vi "ConfigureVirtualChannelModule.vi"(8 "error in (no error)":errorcluster) -> (0 "error out":errorcluster, 1 "register data sets":T1[](array[typedef]), 3 "Virtual Channel Config":T4)   [LabVIEW 2017, in "McsaVirtualChannel.lvlib"]
uses:
  <vilib>/addons/InsightCM/Devices/Shared/Mcsa/McsaVirtualChannel/McsaVirtualChannel.lvlib
  <vilib>/addons/InsightCM/Utilities/GlobalConfiguration/GlobalConfiguration.lvlib
  <vilib>/addons/InsightCM/Utilities/DeviceModelHelpers/DeviceModelHelpers.lvlib
  <vilib>/addons/InsightCM/MessageBus/Base/controls/KeyValuePair.ctl
  <vilib>/addons/InsightCM/MessageBus/Base/controls/Tag.ctl
  <vilib>/addons/InsightCM/Devices/Shared/Mcsa/McsaVirtualChannel/controls/VirtualChannel.ctl
  <vilib>/addons/InsightCM/Devices/Shared/Mcsa/McsaVirtualChannel/controls/VirtualChannelGroup.ctl
  <vilib>/addons/InsightCM/Devices/Shared/Mcsa/McsaVirtualChannel/controls/Config.ctl
  <vilib>/addons/InsightCM/MessageBus/Base/controls/DeviceState.ctl
  <vilib>/addons/InsightCM/MessageBus/Base/controls/Condition.ctl
  <vilib>/addons/InsightCM/MessageBus/Base/controls/Trigger.ctl
  <vilib>/addons/InsightCM/MessageBus/Base/controls/OperatingState.ctl
  <vilib>/addons/InsightCM/MessageBus/Base/controls/R2_DataGroup.ctl
  <vilib>/addons/InsightCM/MessageBus/Base/controls/R2_Device.ctl
  <vilib>/addons/InsightCM/MessageBus/Base/controls/R2_Channel.ctl
  <vilib>/addons/InsightCM/MessageBus/Base/controls/R2_DeviceModel.ctl
  <vilib>/addons/InsightCM/MessageBus/Base/controls/Metric.ctl
  <vilib>/addons/InsightCM/MessageBus/Base/controls/BurstModeTrigger.ctl
  <vilib>/addons/InsightCM/Devices/Shared/Mcsa/McsaDataEventCreator/controls/DataSetType.ctl
  <vilib>/addons/InsightCM/Devices/Shared/Mcsa/McsaDataEventCreator/McsaDataEventCreator.lvlib
  <vilib>/addons/InsightCM/Devices/Shared/Mcsa/McsaDataEventCreator/controls/Registry_DataSet.ctl
  <vilib>/addons/InsightCM/Devices/Shared/Mcsa/McsaDataEventCreator/controls/RegisterDataSets.ctl
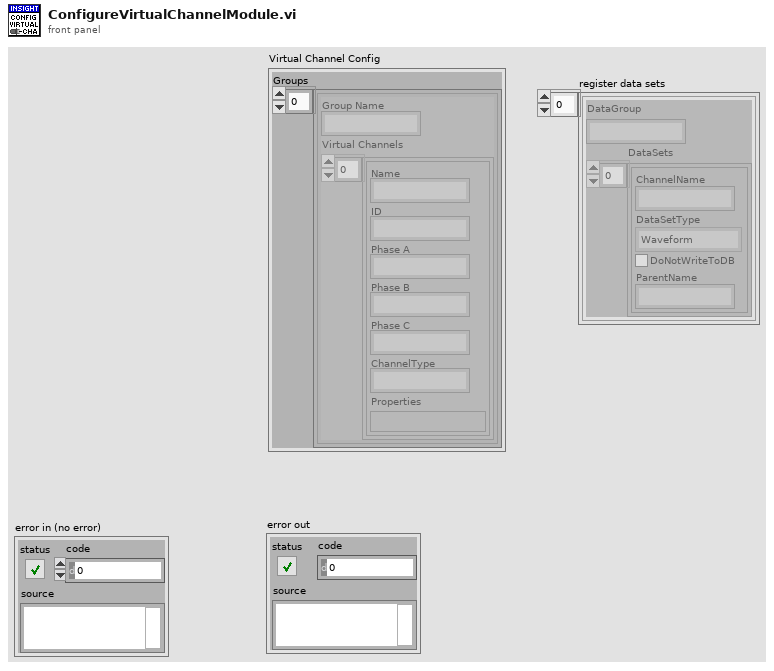
[diagram p1: front panel]
types:
  T1 = typedef "McsaDataEventCreator.lvlib/RegisterDataSets.ctl" = cluster{"DataGroup":string, "DataSets":T2[]}
  T2 = typedef "McsaDataEventCreator.lvlib/Registry_DataSet.ctl" = cluster{"ChannelName":string, "DataSetType":T3, "DoNotWriteToDB":bool, "ParentName":string}
  T3 = typedef "McsaDataEventCreator.lvlib/DataSetType.ctl" = enum16{"Waveform", "MCSAFFT", "TorqueWFM"}
  T4 = typedef "McsaVirtualChannel.lvlib/Config.ctl" = cluster{"Groups":T5[]}
  T5 = typedef "McsaVirtualChannel.lvlib/VirtualChannelGroup.ctl" = cluster{"Group Name":string, "Virtual Channels":T6[]}
  T6 = typedef "McsaVirtualChannel.lvlib/VirtualChannel.ctl" = cluster{"Name":string, "ID":string, "Phase A":string, "Phase B":string, "Phase C":string, "ChannelType":string, "Properties":variant}
  T7 = typedef "R2_DeviceModel.ctl" = cluster{"Device":T8, "Channels":T16[], "Tags":T18[]}
  T8 = typedef "R2_Device.ctl" = cluster{"Id":string, "Name":string, "DeviceType":string, "HardwareName":string, "IpAddress":string, "HardwareInfo":T9[], "ApplicationType":string, "ApplicationVersion":string, "EquipmentIds":string[], "ConfigurationVersion":string, "State":T10, "Properties":T9[], "DataGroups":T11[], "BurstModeTrigger":T15}
  T9 = typedef "KeyValuePair.ctl" = cluster{"Key":string, "Value":string}
  T10 = typedef "DeviceState.ctl" = cluster{"Disabled":bool}
  T11 = typedef "R2_DataGroup.ctl" = cluster{"Name":string, "OperatingStates":T12[], "Properties":T9[], "EquipmentIds":string[], "AssetNodeId":string}
  T12 = typedef "OperatingState.ctl" = cluster{"Name":string, "Properties":T9[], "Triggers":T13[]}
  T13 = typedef "Trigger.ctl" = cluster{"Type":string, "Expression":string, "Conditions":T14[]}
  T14 = typedef "Condition.ctl" = cluster{"Source":string, "Type":string, "Operator":string, "CompareTo":string, "DwellSeconds":dbl}
  T15 = typedef "BurstModeTrigger.ctl" = cluster{"Trigger":T13, "SampleRate":string, "AcquisitionLength":string}
  T16 = typedef "R2_Channel.ctl" = cluster{"Id":string, "DeviceId":string, "Name":string, "ChannelType":string, "HardwareKey":string, "HardwareChannel":string, "DataGroup":string, "Keywords":string[], "EquipmentIds":string[], "Properties":T9[], "Metrics":T17[], "AssetNodeId":string, "MeasType":string, "AssetName":string}
  T17 = typedef "Metric.ctl" = cluster{"Id":string, "Name":string, "Unit":string, "Properties":T9[], "MetricDefinitionInstanceId":string}
  T18 = typedef "Tag.ctl" = cluster{"Id":string, "Path":string, "Name":string, "Datatype":string, "Props":T9[], "Keywords":string[]}
  T19 = typedef "SectionKeyValues.ctl" = cluster{"Section":string, "KeyValues":T9[]}
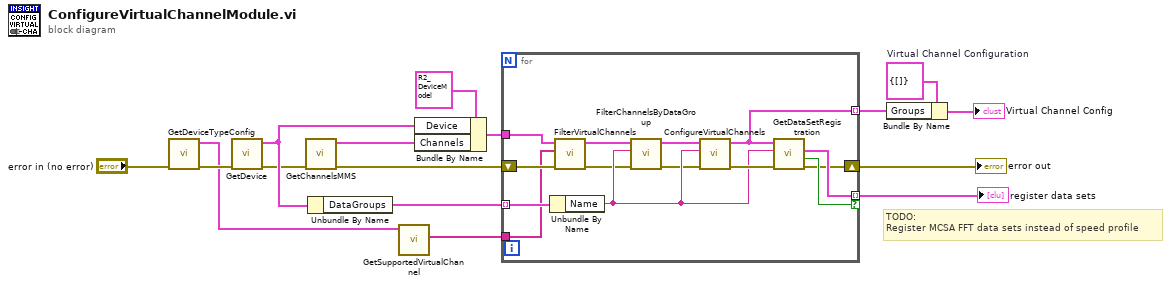
[diagram p0: block diagram]
diagram:
  w8 = T4 {"Groups"=[]}  # Virtual Channel Configuration
  # "TODO:\nRegister MCSA FFT data sets instead of speed profile"
  n1 = call <vilib>:"GetDeviceTypeConfig.vi"("error in (no error)"="error in (no error)") -> ("error out"=w12:errorcluster, "key values"=w7:T19[])  [unwired: 8 in, 1 out]
  n2 = call <vilib>:"GetDevice.vi"("error in (no error)"=w12) -> ("error out"=w1:errorcluster, "device configuration"=w4:T8)  [unwired: 8 in, 1 out]
  n3 = call <vilib>:"GetChannelsMMS.vi"("error in (no error)"=w1) -> ("error out"=w3:errorcluster, "MMS Channels"=w2:T16[])  [unwired: 6 in, 3 out]
  n4 = Unbundle By Name(w4) -> ("DataGroups"=w16:T11[])
  n5 = call <vilib>:"GetSupportedVirtualChannel.vi"("key values"=w7) -> ("not supported virtual channels"=w6:string[])  [unwired: 9 in, 1 out]
  n6 = Bundle By Name(cluster=T7 {"Device"={"Id"="", "Name"="", "DeviceType"="", "HardwareName"="", "IpAddress"="", "HardwareInfo"=[], "ApplicationType"="", "ApplicationVersion"="", "EquipmentIds"=[], "ConfigurationVersion"="", "State"={"Disabled"=FALSE}, "Properties"=[], "DataGroups"=[], "BurstModeTrigger"={"Trigger"={"Type"="", "Expression"="", "Conditions"=[]}, "SampleRate"="", "AcquisitionLength"=""}}, "Channels"=[], "Tags"=[]} ("device model"), "Device"=w4, "Channels"=w2) -> (w9:T7)
  n7 = for {
    shift-right: [w24] -> w15
    shift-left: w3 -> [w21]
    tunnel: w16 -> [w28] mode=indexing
    tunnel: [w29] -> w14 mode=indexing
    tunnel: w6 -> [w19]
    tunnel: w9 -> [w23]
    tunnel: [w26] -> w5 mode=indexing if=w25
    n8 = Unbundle By Name(w28) -> ("Name"=w27:string)
    n9 = call <vilib>:"FilterVirtualChannels.vi"("error in (no error)"=w21, "not supported virtual channels"=w19, "device model"=w23) -> ("error out"=w20:errorcluster, "device model (unsupported virtual channels filtered out)"=w22:T7)  [unwired: 7 in]
    n10 = call <vilib>:"FilterChannelsByDataGroup.vi"("error in (no error)"=w20, "group"=w27, "device model"=w22) -> ("error out"=w17:errorcluster, "channels in data group"=w18:T16[])  [unwired: 7 in]
    n11 = call <vilib>:"ConfigureVirtualChannels.vi"("error in (no error)"=w17, "data group name"=w27, "channels in this group"=w18) -> ("error out"=w30:errorcluster, "virtual channel config"=w29:T5)  [unwired: 6 in, 1 out]
    n12 = call <vilib>:"GetDataSetRegistration.vi"("error in (no error)"=w30, "data group name"=w27, "virtual channel config"=w29) -> ("error out"=w24:errorcluster, "atleast one data set to register"=w25:bool, "register data set"=w26:T1)  [unwired: 6 in]
  }
  "error out" <- w15
  "register data sets" <- w5
  n13 = Bundle By Name(cluster=w8, "Groups"=w14) -> (→"Virtual Channel Config":T4)
